vi "Generate two freq.vi"(5 "input dt":dbl, 7 "samples":i32, 11 "Current treatment":T1) -> (1 "vel":dbl[](array[numeric]), 2 "pos":dbl[](array[numeric]), 3 "Treatment out":T1)   [LabVIEW 2012]
uses:
  Treatment.ctl
  Treatment type.ctl
  <vilib>/Analysis/3filter.llb/Filter Passband Type.ctl
  <vilib>/Analysis/NI_AALBase.lvlib
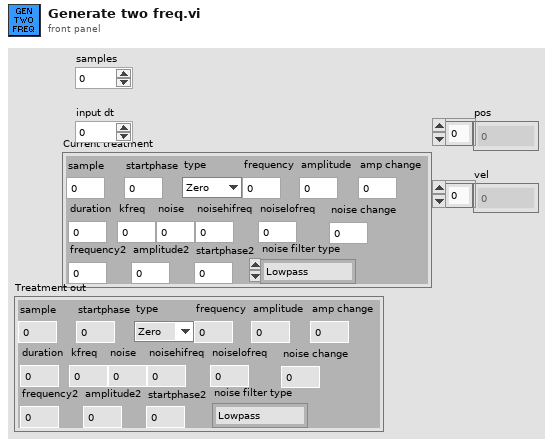
[diagram p1: front panel]
types:
  T1 = typedef "Treatment.ctl" = cluster{"sample":dbl, "startphase":dbl, "type":T2, "frequency":dbl, "amplitude":dbl, "noise":dbl, "duration":dbl, "kfreq":dbl, "noisehifreq":dbl, "frequency2":dbl, "amplitude2":dbl, "startphase2":dbl, "noise filter type":T3, "noiselofreq":dbl, "amp change":dbl, "noise change":dbl}
  T2 = typedef "Treatment type.ctl" = enum16{"Zero", "Sine", "Frequency sweep", "Two frequency"}
  T3 = typedef "NI_AALBase.lvlib/Filter Passband Type.ctl" = enum32{"Lowpass", "Highpass", "Bandpass", "Bandstop"}
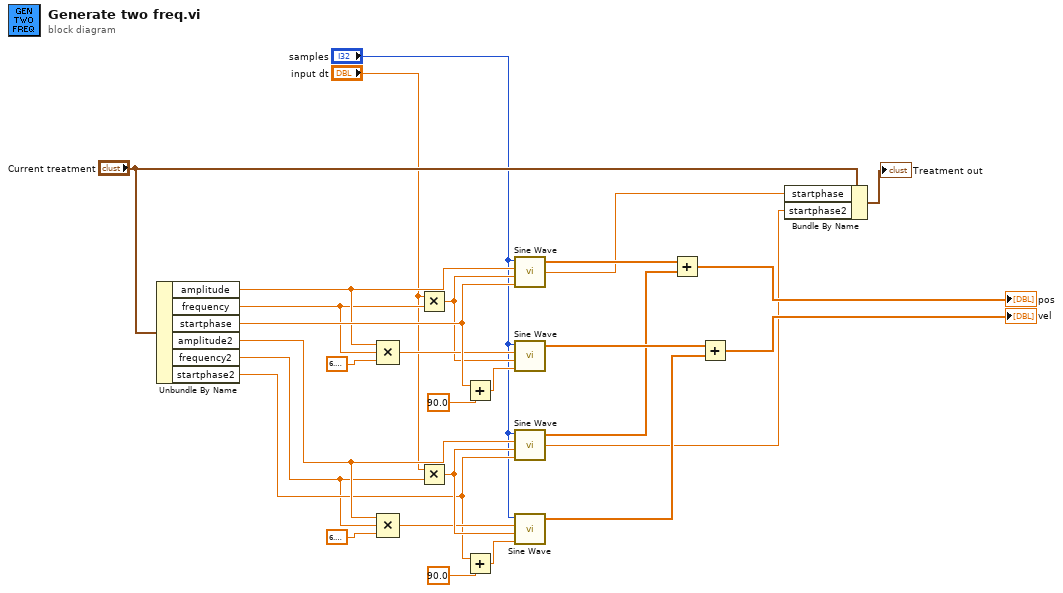
[diagram p0: block diagram]
diagram:
  n1 = Unbundle By Name("Current treatment") -> ("amplitude"=w27:dbl, "frequency"=w24:dbl, "startphase"=w28:dbl, "amplitude2"=w8:dbl, "frequency2"=w6:dbl, "startphase2"=w7:dbl)
  n2 = Compound Arithmetic op=MULTIPLY(w27, w24, 6.283185307179586) -> (w22:dbl)
  n3 = Compound Arithmetic op=MULTIPLY(w8, w6, 6.283185307179586) -> (w10:dbl)
  n4 = Multiply(x="input dt", y=w24) -> (x*y=w20:dbl)
  n5 = Multiply(x="input dt", y=w6) -> (x*y=w11:dbl)
  n6 = Add(x=w28, y=90.0) -> (x+y=w18:dbl)
  n7 = Add(x=w7, y=90.0) -> (x+y=w12:dbl)
  n8 = call <vilib>:"Sine Wave.vi"("samples"="samples", "amplitude"=w27, "frequency"=w20, "phase in"=w28) -> ("sine wave"=w19:dbl[], "phase out"=w15:dbl)  [unwired: 1 in, 1 out]
  n9 = call <vilib>:"Sine Wave.vi"("samples"="samples", "amplitude"=w22, "frequency"=w20, "phase in"=w18) -> ("sine wave"=w21:dbl[])  [unwired: 1 in, 2 out]
  n10 = call <vilib>:"Sine Wave.vi"("samples"="samples", "amplitude"=w8, "frequency"=w11, "phase in"=w7) -> ("sine wave"=w3:dbl[], "phase out"=w1:dbl)  [unwired: 1 in, 1 out]
  n11 = call <vilib>:"Sine Wave.vi"("samples"="samples", "amplitude"=w10, "frequency"=w11, "phase in"=w12) -> ("sine wave"=w2:dbl[])  [unwired: 1 in, 2 out]
  n12 = Add(x=w19, y=w3) -> (x+y=→"pos":dbl[])
  n13 = Add(x=w21, y=w2) -> (x+y=→"vel":dbl[])
  n14 = Bundle By Name(cluster="Current treatment", "startphase"=w15, "startphase2"=w1) -> (→"Treatment out":T1)
